vi "SV Configure Generator.vi"   [LabVIEW 2017, in "SV Signal.lvclass"]
doc: "Configures a user-defined test signal. Wire the outputs to SV Signal (waveform) VI to generate the test signal, or wire to SV Signal Property Node to configure additional parameters before wiring to the SV Signal (waveform) VI."
uses:
  <vilib>/addons/_NISVFA/_Generation/Signal Generation/SV Signal/SV Signal.lvclass
  <vilib>/addons/_NISVFA/_Generation/Signal Generation/SV Sinusoid/SV Sinusoid.lvclass
  <vilib>/addons/_NISVFA/_Generation/Signal Generation/SV Square/SV Square.lvclass
  <vilib>/addons/_NISVFA/_Generation/Signal Generation/SV Triangle/SV Triangle.lvclass
  <vilib>/addons/_NISVFA/_Generation/Signal Generation/SV Noise/SV Noise.lvclass
  <vilib>/addons/_NISVFA/_Generation/Signal Generation/SV MLS/SV MLS.lvclass
  <vilib>/addons/_NISVFA/_Generation/Signal Generation/SV Multitone/SV Multitone.lvclass
  <vilib>/addons/_NISVFA/_Generation/Signal Generation/SV Continuous Sweep/SV Continuous Sweep.lvclass
  <vilib>/addons/_NISVFA/_Generation/Signal Generation/SV Discrete Sweep/SV Discrete Sweep.lvclass
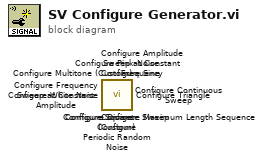
[diagram p0: block diagram]
diagram:
  n1 = call <vilib>:"Configure Discrete Sweep (Custom).vi"() -> ()  [unwired: 14 in, 2 out]
  n2 = call <vilib>:"Configure Amplitude Sweep at Constant Frequency.vi"() -> ()  [unwired: 14 in, 2 out]
  n3 = call <vilib>:"Configure Frequency Sweep at Constant Amplitude.vi"() -> ()  [unwired: 14 in, 2 out]
  n4 = call <vilib>:"Configure Continuous Sweep.vi"() -> ()  [unwired: 14 in, 2 out]
  n5 = call <vilib>:"Configure Multitone (Custom).vi"() -> ()  [unwired: 13 in, 3 out]
  n6 = call <vilib>:"Configure Maximum Length Sequence.vi"() -> ()  [unwired: 14 in, 2 out]
  n7 = call <vilib>:"Configure Periodic Random Noise.vi"() -> ()  [unwired: 14 in, 2 out]
  n8 = call <vilib>:"Configure Pink Noise.vi"() -> ()  [unwired: 14 in, 2 out]
  n9 = call <vilib>:"Configure White Noise.vi"() -> ()  [unwired: 14 in, 2 out]
  n10 = call <vilib>:"Configure Triangle.vi"() -> ()  [unwired: 14 in, 2 out]
  n11 = call <vilib>:"Configure Square.vi"() -> ()  [unwired: 14 in, 2 out]
  n12 = call <vilib>:"Configure Sine.vi"() -> ()  [unwired: 14 in, 2 out]
